vi "cristains openQCM filter.vi"() -> ()   [LabVIEW 2014]
uses:
  <vilib>/Analysis/baseanly.llb/Mean (DBL).vi
  <vilib>/Instr/_visa.llb/VISA Configure Serial Port (Instr).vi
  <vilib>/Utility/file.llb/Write To Spreadsheet File (string).vi
  <vilib>/Analysis/NI_AALBase.lvlib
panel:
  in  "error in (no error)":errorcluster
  out "error out":errorcluster
  out "Temp (K)":dbl
  in  "Arduino address":refnum<visa-resource-name>
  out "Waveform Chart":cluster{dbl, "mean":dbl, "median":dbl}(graph)
  in  "Stop Button":bool
  out "Median (Hz)":dbl format="%#_8g"
  out "Mean (Hz)":dbl format="%#_8g"
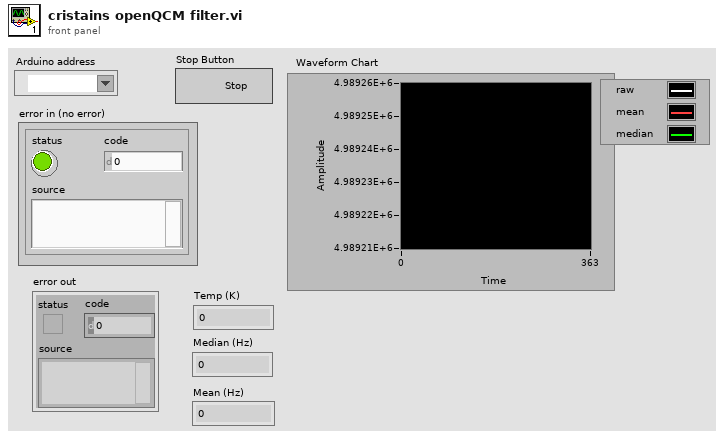
[diagram p1: front panel]
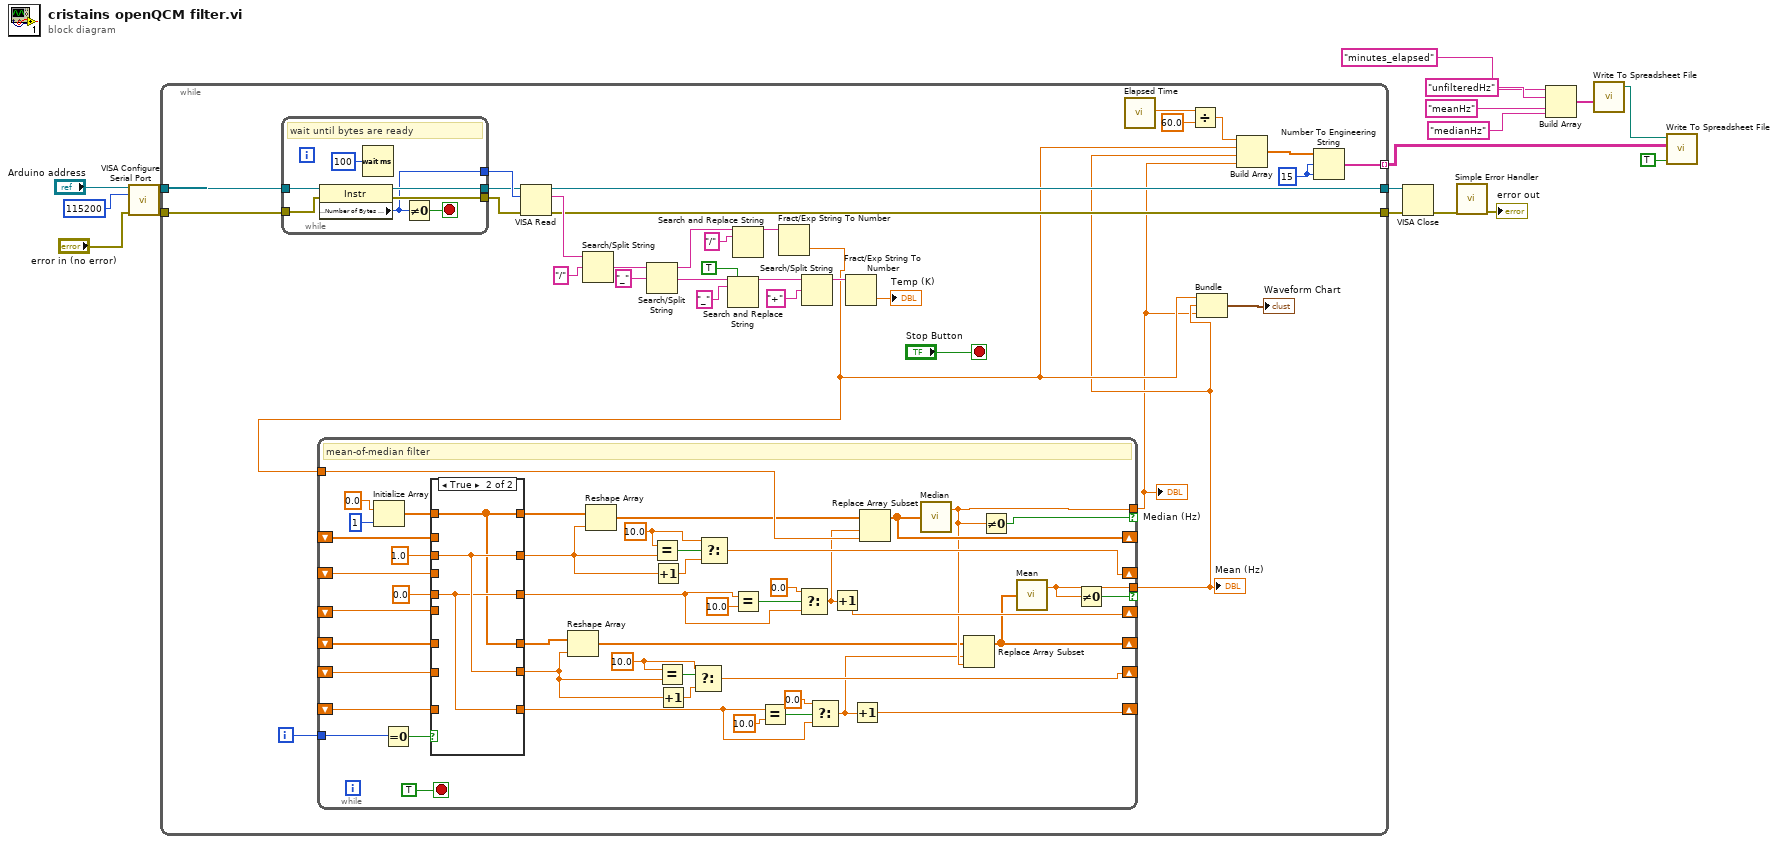
[diagram p0: block diagram]
diagram:
  n1 = call-poly "VISA Configure Serial Port"("VISA resource name"="Arduino address", "baud rate (9600)"=u32 115200, "error in (no error)"="error in (no error)") -> ("VISA resource name out"=w14:refnum<visa-resource-name>, "error out"=w13:errorcluster)  [unwired: 11 in]
  n2 = while {
    tunnel: w14 -> [w30]
    tunnel: w13 -> [w29]
    tunnel: [w28] -> w10
    tunnel: [w27] -> w9
    tunnel: [w18] -> w2 mode=indexing
    i -> [w49]
    stop <- "Stop Button" stop-if-true
    w26 = i16 15 ("width (-)")
    n3 = while {
      tunnel: w29 -> [w56]
      tunnel: w30 -> [w57]
      tunnel: [w55] -> w32
      tunnel: [w54] -> w31
      tunnel: [w53] -> w33
      stop <- w51 stop-if-true
      # "wait until bytes are ready"
      n4 = property class="Instr"(reference=w57, error in=w56) -> (reference out=w54:refnum<visa-resource-name>, error out=w55:errorcluster, "Serial Settings:Number of Bytes at Serial Port"=w53:u32)
      n5 = Wait (ms)(milliseconds to wait=u32 100) -> ()  [unwired: 1 out]
      n6 = Not Equal To 0?(x=w53) -> (x != 0?=w51:bool)
    }
    n7 = VISA Read(VISA resource name=w31, byte count=w33, error in (no error)=w32) -> (VISA resource name out=w28:refnum<visa-resource-name>, read buffer=w47:string, error out=w27:errorcluster)  [unwired: 1 out]
    n8 = Search/Split String(string=w47, search string/char (-)="/") -> (match + rest of string=w39:string)  [unwired: 1 in, 2 out]
    n9 = Search/Split String(string=w39, search string/char (-)="_") -> (substring before match=w45:string, match + rest of string=w40:string)  [unwired: 1 in, 1 out]
    n10 = Search and Replace String(replace all?=TRUE ("replace all? (F)"), input string=w40, search string="_") -> (result string=w34:string)  [unwired: 5 in, 3 out]
    n11 = Search and Replace String(input string=w45, search string="/" ("replace string (\"\")")) -> (result string=w36:string)  [unwired: 6 in, 3 out]
    n12 = Fract/Exp String To Number(string=w36) -> (number=w21:dbl)  [unwired: 3 in, 1 out]
    n13 = while {
      shift-right: [w96] -> _
      shift-left: _ -> [w74]
      shift-right: [w104] -> _
      shift-left: _ -> [w67]
      shift-right: [w93] -> _
      shift-left: _ -> [w64]
      shift-right: [w103] -> _
      shift-left: _ -> [w60]
      shift-right: [w102] -> _
      shift-left: _ -> [w71]
      tunnel: w21 -> [w99]
      tunnel: w49 -> [w76]
      tunnel: [w95] -> w20 if=w98
      tunnel: [w92] -> w19 if=w91
      shift-right: [w94] -> _
      shift-left: _ -> [w62]
      stop <- TRUE stop-if-true
      w77 = 10.0 ("t")
      w69 = 10.0 ("y")
      # "mean-of-median filter"
      n14 = Initialize Array(0.0 ("element"), 1 ("dimension size")) -> (w65:dbl[])
      n15 = Equal To 0?(x=w76) -> (x = 0?=w75:bool)
      n16 = case shown="True" w75 {
        tunnel: w65 -> [_ w111]
        tunnel: w74 -> [w110 _]
        tunnel: [w110 w111] -> w73
        tunnel: 1.0 ("t") -> [_ w113]
        tunnel: w71 -> [w109 _]
        tunnel: [w109 w113] -> w70
        tunnel: 0.0 ("t") -> [_ w112]
        tunnel: [w108 w112] -> w66
        tunnel: w67 -> [w108 _]
        tunnel: [w107 w111] -> w63
        tunnel: w64 -> [w107 _]
        tunnel: [w106 w113] -> w61
        tunnel: w62 -> [w106 _]
        tunnel: w60 -> [w105 _]
        tunnel: [w105 w112] -> w59
        frame False {
        }
        frame True {
        }
      }
      n17 = Reshape Array(w63, w61) -> (w58:dbl[])
      n18 = Reshape Array(w73, w70) -> (w84:dbl[])
      n19 = Equal?(x=w69, y=w70) -> (x = y?=w83:bool)
      n20 = Increment(x=w70) -> (x+1=w82:dbl)
      n21 = Equal?(x=w77, y=w61) -> (x = y?=w80:bool)
      n22 = Increment(x=w61) -> (x+1=w79:dbl)
      n23 = Select(t=w77, s=w80, f=w79) -> (s? t:f=w94:dbl)
      n24 = Select(t=w69, s=w83, f=w82) -> (s? t:f=w102:dbl)
      n25 = Equal?(x=w66, y=10.0) -> (x = y?=w90:bool)
      n26 = Equal?(x=w59, y=10.0) -> (x = y?=w87:bool)
      n27 = Select(t=0.0, s=w90, f=w66) -> (s? t:f=w78:dbl)
      n28 = Select(t=0.0, s=w87, f=w59) -> (s? t:f=w86:dbl)
      n29 = Increment(x=w78) -> (x+1=w104:dbl)
      n30 = Increment(x=w86) -> (x+1=w103:dbl)
      n31 = Replace Array Subset(array=w84, new element=w99, index=w78) -> (w96:dbl[])
      n32 = call <vilib>:"Median.vi"("X"=w96) -> ("median"=w92:dbl)  [unwired: 1 out]
      n33 = Replace Array Subset(array=w58, new element=w92, index=w86) -> (w93:dbl[])
      n34 = Not Equal To 0?(x=w92) -> (x != 0?=w91:bool)
      n35 = call-poly <vilib>:"Mean.vi"("X"=w93) -> ("mean"=w95:dbl)  [unwired: 1 out]
      n36 = Not Equal To 0?(x=w95) -> (x != 0?=w98:bool)
    }
    "Mean (Hz)" <- w20
    "Median (Hz)" <- w19
    n37 = Search/Split String(string=w34, search string/char (-)="+") -> (substring before match=w43:string)  [unwired: 1 in, 2 out]
    n38 = Fract/Exp String To Number(string=w43) -> (number=→"Temp (K)":dbl)  [unwired: 3 in, 1 out]
    n39 = call "Elapsed Time"() -> ("Elapsed Time (s)"=w22:dbl)  [unwired: 12 in, 7 out]
    n40 = Divide(x=w22, y=60.0) -> (x/y=w25:dbl)
    n41 = Bundle(w21, "mean"=w20, "median"=w19) -> (→"Waveform Chart":cluster{dbl, "mean":dbl, "median":dbl})  [unwired: 1 in]
    n42 = Build Array(w25, w21, w20, w19) -> (w24:dbl[])
    n43 = Number To Engineering String(2:w26, 3:w26, 4:w24) -> (0:w18:string[])  [unwired: 1 in]
  }
  n44 = VISA Close(VISA resource name=w10, error in (no error)=w9) -> (error out=w11:errorcluster)
  n45 = call <vilib>:"Simple Error Handler.vi"("error in (no error)"=w11) -> ("error out"=→"error out":errorcluster)  [unwired: 4 in, 4 out]
  n46 = Build Array("minutes_elapsed" ("element"), "unfilteredHz", "meanHz", "medianHz") -> (w7:string[])
  n47 = call-poly <vilib>:"Write To Spreadsheet File.vi"("1D data"=w7) -> ("new file path (Not A Path if cancelled)"=w6:path)  [unwired: 7 in]
  n48 = call-poly <vilib>:"Write To Spreadsheet File.vi"("append to file? (new file:F)"=TRUE ("transpose? (no:F)"), "2D data"=w2, "file path (dialog if empty)"=w6) -> ()  [unwired: 5 in, 1 out]
